vi "MCAData.vi"(8 "error in":errorcluster, 10 "CrsrList":T2) -> (0 "error out":errorcluster, 1 "MCA Out":T1, 2 "Spectrum":u32[][](array[numeric]))   [LabVIEW 2011]
uses:
  <vilib>/Utility/miscctls.llb/LVCursorListTypeDef.ctl
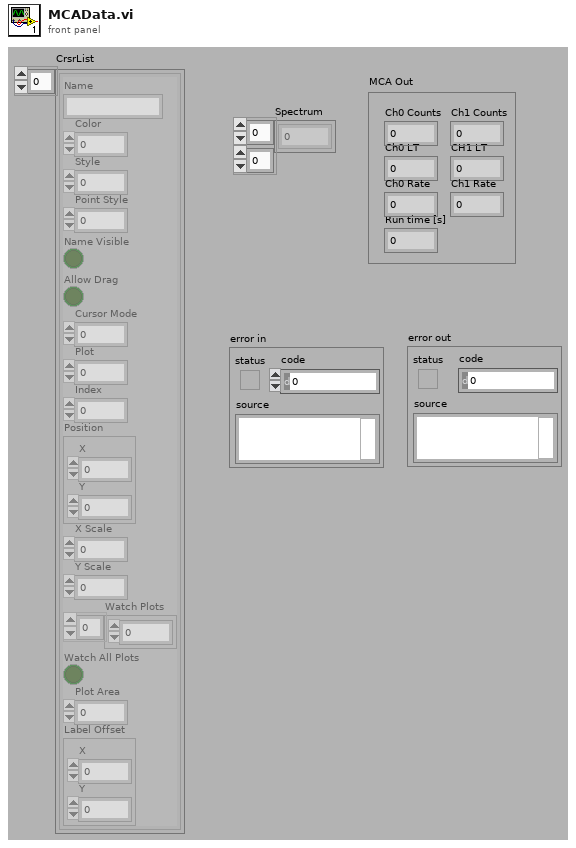
[diagram p1: front panel]
types:
  T1 = cluster{"Ch0 Counts":u32, "Ch0 Rate":dbl, "Ch1 Counts":u32, "Ch1 Rate":dbl, "Ch0 LT":dbl, "CH1 LT":dbl, "Run time [s]":dbl}
  T2 = typedef "LVCursorListTypeDef.ctl" = cluster{"Name":string, "Color":u32, "Style":u8, "Point Style":u8, "Name Visible":bool, "Allow Drag":bool, "Cursor Mode":u32, "Plot":i32, "Index":i32, "Position":cluster{"X":dbl, "Y":dbl}, "X Scale":u32, "Y Scale":u32, "Watch Plots":i32[], "Watch All Plots":bool, "Plot Area":i32, "Label Offset":cluster{"X":dbl, "Y":dbl}}[]
  T3 = cluster{"Name":string, "Color":u32, "Style":u8, "Point Style":u8, "Name Visible":bool, "Allow Drag":bool, "Cursor Mode":u32, "Plot":i32, "Index":i32, "Position":cluster{"X":dbl, "Y":dbl}, "X Scale":u32, "Y Scale":u32, "Watch Plots":i32[], "Watch All Plots":bool, "Plot Area":i32, "Label Offset":cluster{"X":dbl, "Y":dbl}}
  T4 = cluster{"Ch0 Counts":u32, "Ch0 Rate":dbl, "Ch1 Counts":u32, "Ch1 Rate":dbl, "livetime":dbl, "livetime":dbl, "Run time [s]":dbl}
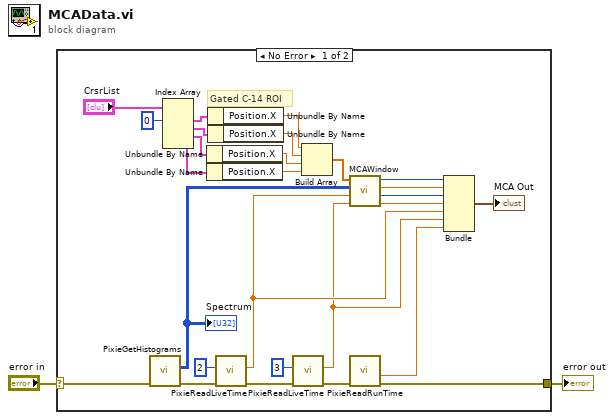
[diagram p0: block diagram]
diagram:
  n1 = case shown="No Error" "error in" {
    selector: "error in" -> [w11 w30]
    tunnel: [w12 w30] -> w2
    frame No Error {
      # "Gated C-14 ROI"
      n2 = call "PixieGetHistograms.vi"("error in (no error)"=w11) -> ("error out"=w13:errorcluster, "Histogram Data"=w29:u32[][])  [unwired: 1 in, 8 out]
      "Spectrum" <- w29
      n3 = Index Array(array="CrsrList", index #1=0 ("index")) -> (element #1=w19:T3, element #2=w18:T3, element #3=w17:T3, element #4=w16:T3)  [unwired: 3 in]
      n4 = Unbundle By Name(w17) -> ("Position.X"=w28:dbl)
      n5 = Unbundle By Name(w16) -> ("Position.X"=w24:dbl)
      n6 = Unbundle By Name(w19) -> ("Position.X"=w22:dbl)
      n7 = Unbundle By Name(w18) -> ("Position.X"=w23:dbl)
      n8 = call "PixieReadLiveTime.vi"("error in (no error)"=w13, "ChanNum"=u16 2) -> ("error out"=w14:errorcluster, "livetime"=w6:dbl)  [unwired: 8 out]
      n9 = call "PixieReadLiveTime.vi"("error in (no error)"=w14, "ChanNum"=u16 3) -> ("error out"=w27:errorcluster, "livetime"=w5:dbl)  [unwired: 8 out]
      n10 = Build Array(w22, w23, w28, w24) -> (w25:dbl[])
      n11 = call "MCAWindow.vi"("Ch1 Livetime"=w5, "Ch0 Livetime"=w6, "Histogram Data"=w29, "Window"=w25) -> ("Ch1 Rate"=w7:dbl, "Ch1 Counts"=w8:u32, "Ch0 Rate"=w9:dbl, "Ch0 Counts"=w10:u32)  [unwired: 4 out]
      n12 = call "PixieReadRunTime.vi"("error in (no error)"=w27) -> ("error out"=w12:errorcluster, "Run time [s]"=w4:dbl)  [unwired: 1 in, 8 out]
      n13 = Bundle("Ch0 Counts"=w10, "Ch0 Rate"=w9, "Ch1 Counts"=w8, "Ch1 Rate"=w7, "livetime"=w6, "livetime"=w5, "Run time [s]"=w4) -> (→"MCA Out":T4)  [unwired: 1 out]
    }
    frame Error {
    }
  }
  "error out" <- w2
